vi "Write Initialized Status.vi"   [LabVIEW 2023, in "Cycler.lvclass"]
uses:
  Cycler.lvclass
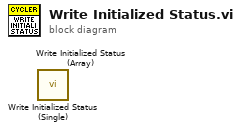
[diagram p0: block diagram]
diagram:
  n1 = call "Write Initialized Status (Single).vi"() -> ()  [unwired: 10 in, 2 out]
  n2 = call "Write Initialized Status (Array).vi"() -> ()  [unwired: 10 in, 2 out]
